vi "Add APU.vi"(8 "error in (no error)":errorcluster, 10 "APU name":string, 11 "EST custom device in":refnum<k24>) -> (0 "error out":errorcluster, 2 "APU Node":refnum<k24>, 3 "EST custom device out":refnum<k24>)   [LabVIEW 2015, in "Engine Simulation Toolkit SysDef API.lvlib"]
uses:
  Engine Simulation Toolkit SysDef API.lvlib
  NationalInstruments.VeriStand.SystemDefinitionAPI
  System Explorer/Engine Simulation Toolkit System Explorer.lvlib
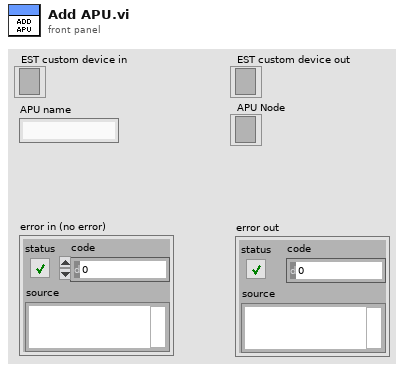
[diagram p1: front panel]
types:
  T1 = typedef "Custom Device API.lvlib/Custom Device Item Ref.ctl" = u64
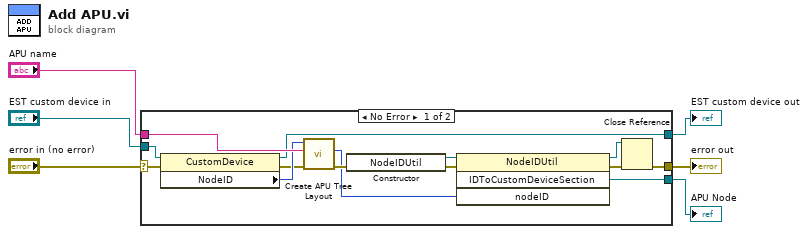
[diagram p0: block diagram]
diagram:
  n1 = case shown="No Error" "error in (no error)" {
    selector: "error in (no error)" -> [w18 w22]
    tunnel: "APU name" -> [w20 _]
    tunnel: "EST custom device in" -> [w19 w21]
    tunnel: [w16 w21] -> w4
    tunnel: [w9 w22] -> w3
    tunnel: [w7 _] -> w1
    frame No Error {
      n2 = property class="CustomDevice"(reference=w19, error in=w18) -> (reference out=w16:refnum<k24>, error out=w15:errorcluster, "NodeID"=w17:u64)
      n3 = call "Create APU Tree Layout.vi"("error in (no error)"=w15, "engine name"=w20, "Section Ptr"=w17) -> ("error out"=w10:errorcluster, "APU ref"=w8:T1)  [unwired: 6 in, 1 out]
      n4 = constructor class="NodeIDUtil"(error in=w10) -> (reference out=w11:refnum<k24>, error out=w12:errorcluster)  [unwired: 2 in, 1 out]
      n5 = invoke class="NodeIDUtil" method="IDToCustomDeviceSection"(reference=w11, error in=w12, "nodeID"=w8) -> (reference out=w13:refnum<k24>, error out=w14:errorcluster, "IDToCustomDeviceSection"=w7:refnum<k24>)  [unwired: 1 in, 1 out]
      n6 = Close Reference(reference=w13, error in (no error)=w14) -> (error out=w9:errorcluster)
    }
    frame Error {
    }
  }
  "APU Node" <- w1
  "EST custom device out" <- w4
  "error out" <- w3
